vi "Get Command Field Width.vi"(8 "error in (no error)":errorcluster, 11 "RFFE Command in":refnum<class "RFFE Command.lvclass">) -> (0 "error out":errorcluster, 2 "Command Field Width":i32, 3 "RFFE Command out":refnum<class "RFFE Command.lvclass">)   [LabVIEW 2018, in "MIPI RFFE API.lvlib" / "RFFE Command.lvclass"]
uses:
  RFFE Command.lvclass
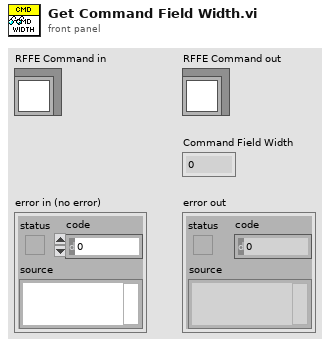
[diagram p1: front panel]
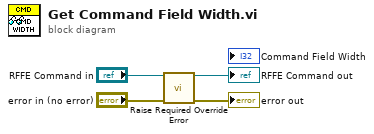
[diagram p0: block diagram]
diagram:
  n1 = call "Raise Required Override Error.vi"("RFFE Command in"="RFFE Command in", "error in (no error)"="error in (no error)") -> ("RFFE Command out"=→"RFFE Command out":refnum<class "RFFE Command.lvclass">, "error out"=→"error out":errorcluster)  [unwired: 11 in, 1 out]
